vi "Boolean to String.vi"(10 "Boolean":bool) -> (2 "String":string)   [LabVIEW 2013]
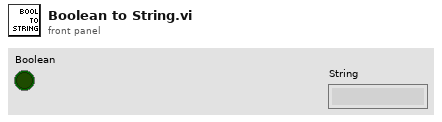
[diagram p1: front panel]
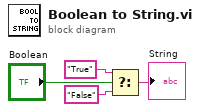
[diagram p0: block diagram]
diagram:
  n1 = Select(t="True", s="Boolean", f="False") -> (s? t:f=→"String":string)
